vi "mouse.vi"() -> ()   [LabVIEW 2016]
uses:
  <vilib>/Utility/inputDevices.llb/mouseAcquire.vi
  <vilib>/Utility/inputDevices.llb/closeMouse.vi
panel:
  out "button info":T1
  out "axis info":T2
  in  "Stop Button":bool
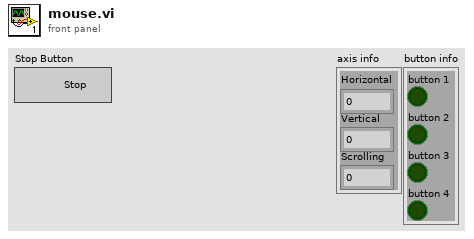
[diagram p1: front panel]
types:
  T1 = cluster{"button 1":bool, "button 2":bool, "button 3":bool, "button 4":bool}
  T2 = cluster{"Horizontal":i32, "Vertical":i32, "Scrolling":i32}
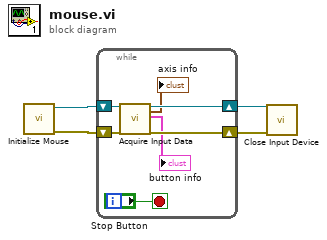
[diagram p0: block diagram]
diagram:
  n1 = call <vilib>:"Initialize Mouse.vi"() -> ("error out"=w4:errorcluster, "device ID"=w3:refnum<k1>)  [unwired: 10 in]
  n2 = while {
    shift-right: [w9] -> w2
    shift-left: w4 -> [w11]
    shift-right: [w8] -> w1
    shift-left: w3 -> [w10]
    stop <- "Stop Button" stop-if-true
    n3 = call-poly <vilib>:"Acquire Input Data.vi"("device ID"=w10, "error in (no error)"=w11) -> ("device ID"=w8:refnum<k1>, "axis info"=→"axis info":T2, "button info"=→"button info":T1, "error out"=w9:errorcluster)  [unwired: 14 in]
  }
  n4 = call-poly <vilib>:"Close Input Device.vi"("error in (no error)"=w2, "device ID"=w1) -> ()  [unwired: 8 in, 1 out]
